vi "mtoe far.vi"(11 "m":dbl) -> (3 "e":dbl)   [LabVIEW 2019]
panel:
  in  "y":dbl=9280.4 format="%#_13g"
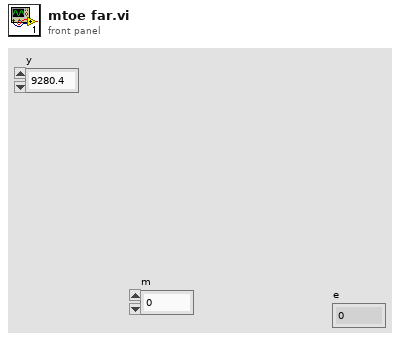
[diagram p1: front panel]
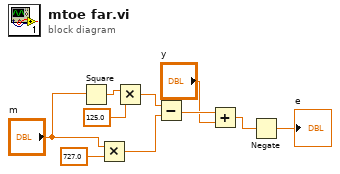
[diagram p0: block diagram]
diagram:
  n1 = Square(x="m") -> (x^2=w10:dbl)
  n2 = Multiply(x="m", y=727.0) -> (x*y=w5:dbl)
  n3 = Multiply(x=w10, y=125.0) -> (x*y=w8:dbl)
  n4 = Subtract(x=w8, y=w5) -> (x-y=w4:dbl)
  n5 = Add(x=w4, y="y") -> (x+y=w3:dbl)
  n6 = Negate(x=w3) -> (-x=→"e":dbl)
